vi "Write PhaseRange.vi"(8 "error in (no error)":errorcluster, 10 "PhaseRange":u16[](array[numeric]), 11 "CorrFactor in":refnum<class "CorrFactor.lvclass">) -> (0 "error out":errorcluster, 3 "CorrFactor out":refnum<class "CorrFactor.lvclass">)   [LabVIEW 2018, in "AnalysisPlugins.lvlib" / "CorrFactor.lvclass"]
uses:
  CorrFactor.lvclass
  CorrFactor.lvclass/CorrFactor.ctl
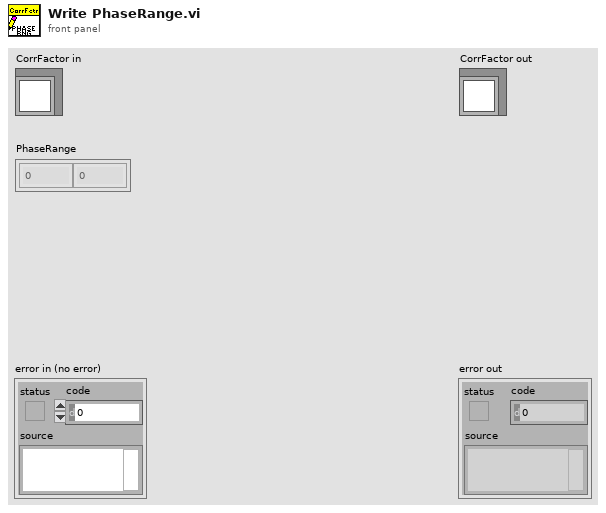
[diagram p1: front panel]
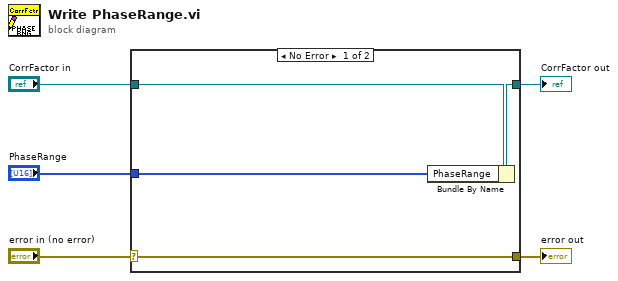
[diagram p0: block diagram]
diagram:
  n1 = case shown="No Error" "error in (no error)" {
    selector: "error in (no error)" -> [w9 w10]
    tunnel: [w9 w10] -> w4
    tunnel: [w7 w11] -> w2
    tunnel: "CorrFactor in" -> [w8 w11]
    tunnel: "PhaseRange" -> [w6 _]
    frame No Error {
      n2 = Bundle By Name(cluster=w8, "PhaseRange"=w6) -> (w7:refnum<class "CorrFactor.lvclass">)
    }
    frame Error {
    }
  }
  "error out" <- w4
  "CorrFactor out" <- w2
